vi "LED Controller.vi"(8 "error in":errorcluster) -> ()   [LabVIEW 2023]
doc: "This VI executes continuously carrying out the current operation and responding to updates or new operations. It will often contain the timing or control code that is difficult to place directly in TeleOp. This VI generally opens all sensors and motors and isolates the rest of the robot code from knowing how the operations are carried out."
uses:
  <vilib>/Rock Robotics/WPI/Framework/Completion Status.ctl
  LED Setpoints.ctl
  LED Operations.ctl
  source files/Amp-Speaker.ctl
  source files/Lights Setpoints.ctl
  <vilib>/Rock Robotics/SystemInterfaces/DIO/FPGA_DIOPWMChannel.ctl
  source files/ArduinoSerialBling.lvlib
  <vilib>/Rock Robotics/Network Tables/NT Write Boolean.vi
panel:
  in  "Blending LEDs":u8=21
  in  "String Length":u16=21
  in  "Interactive Values":T1
  out "Current\nCmd":string
  in  "Buttons":cluster{"Execute Cmd":bool, "Abort Cmd":bool}
  out "Command Timing":cluster{"Start Time (ms)":u32, "Iterations":i32}
  out "Status":T5
  # "Tip: It may be helpful to observe inputs and sensor values.\nYou may also want to display tuning or debugging controls."
  # "Interactive Command: You may fill in the settings for a command\nand schedule it with the Execute button. You can observe and abort\nany command while fine tuning the code for the controller."
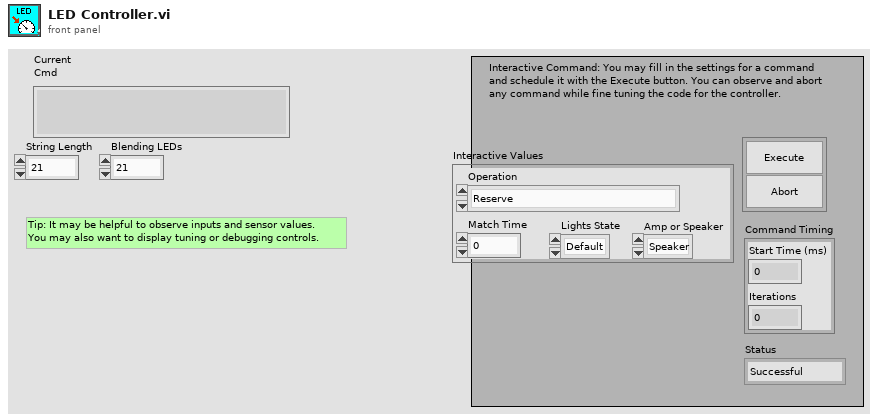
[diagram p1: front panel]
types:
  T1 = typedef "LED Setpoints.ctl" = cluster{"Operation":T2, "Match Time":dbl, "Lights State":T3, "Amp or Speaker":T4}
  T2 = typedef "LED Operations.ctl" = enum16{"Reserve", "Read Current", "Immediate"}
  T3 = typedef "Amp-Speaker.ctl" = enum16{"Default", "Flywheel State", "Endgame", "Note Detection"}
  T4 = typedef "Lights Setpoints.ctl" = enum16{"Speaker", "Amp"}
  T5 = typedef "Completion Status.ctl" = enum16{"Successful", "Aborted", "Incomplete"}
  T6 = typedef "FPGA_DIOPWMChannel.ctl" = enum8{"PWM 0", "PWM 1", "PWM 2", "PWM 3", "PWM 4", "PWM 5", "PWM 6", "PWM 7", "PWM 8", "PWM 9", "PWM MXP 0", "PWM MXP 1", "PWM MXP 2", "PWM MXP 3", "PWM MXP 4", "PWM MXP 5", "PWM MXP 6", "PWM MXP 7", "PWM MXP 8", "PWM MXP 9", "Invalid"}
  T7 = typedef "WPI_PWMDeviceRef.ctl" = cluster{"DeviceStatus":errorcluster, "PWM Channel":T6}
  T8 = typedef "Command Status Info.ctl" = cluster{"Name":string, "Status":T5, "notifier out":T9}
  T9 = typedef "Completion Notifier.ctl" = refnum<notifier>
  T10 = cluster{"Current Command":T1, "Command Timing":cluster{"Start Time (ms)":u32, "Iterations":i32}, "Command Arguments":cluster{"Command Info":T8, "Description":string, "Default Command":T1, "queue out":refnum<queue>, "Subsystem Name":string}}
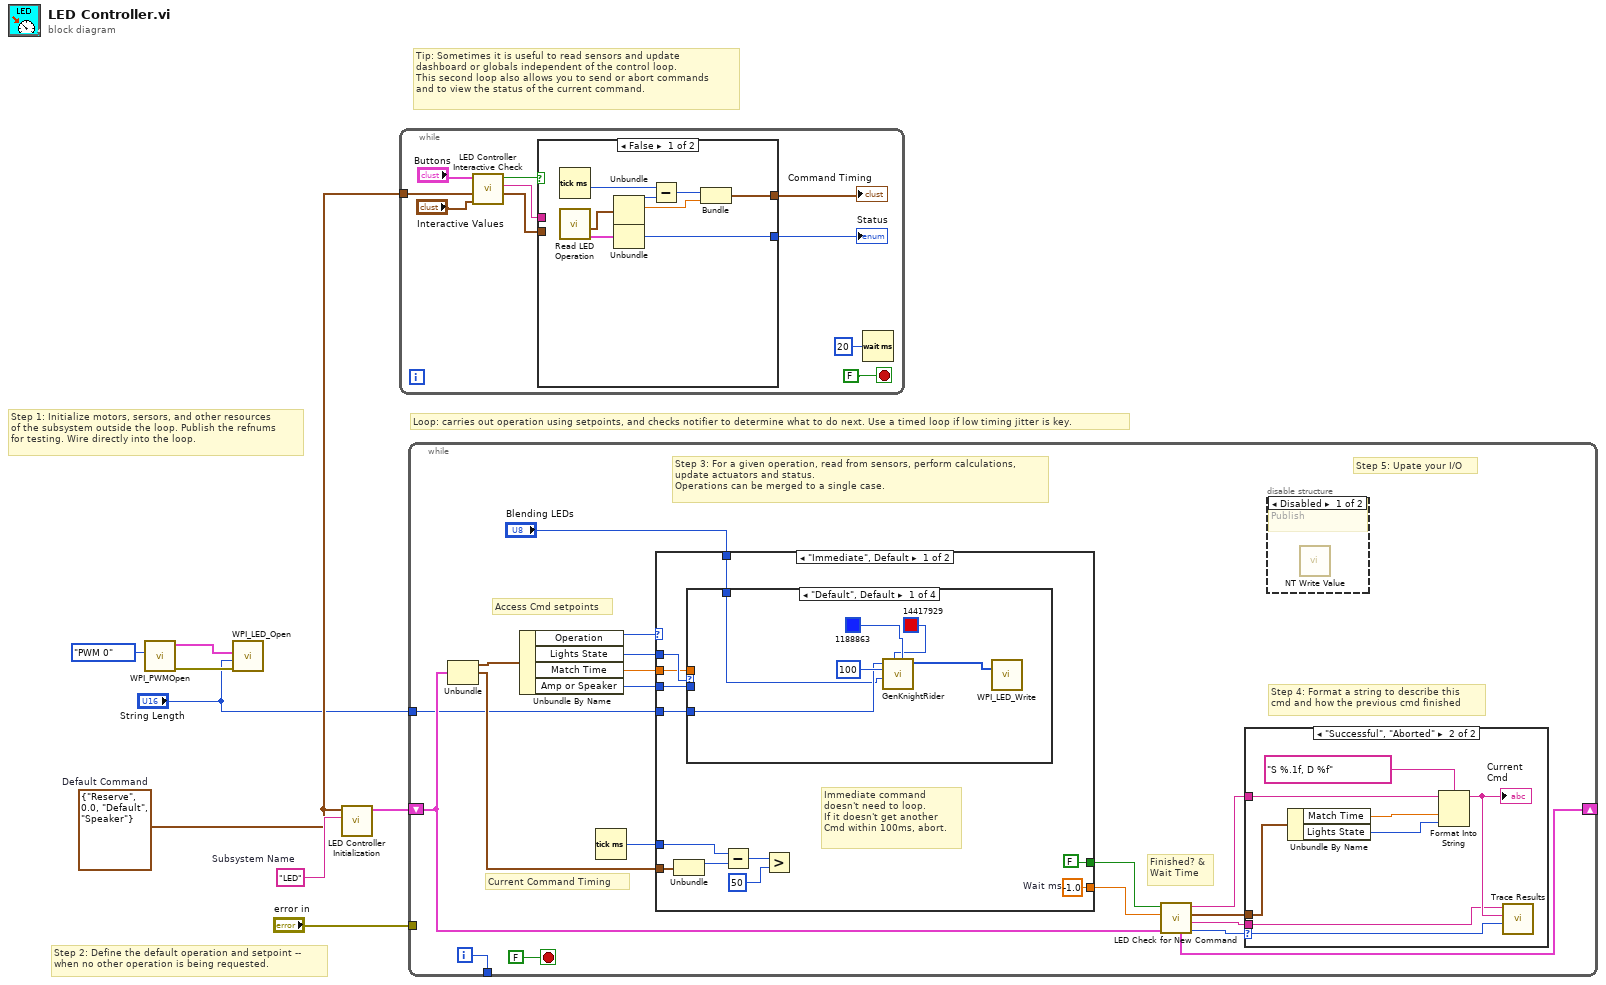
[diagram p0: block diagram]
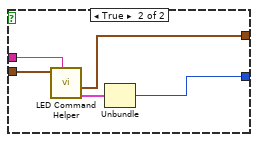
[diagram p2: hidden frame]
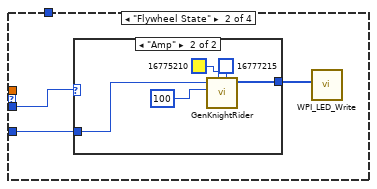
[diagram p5: hidden frame]
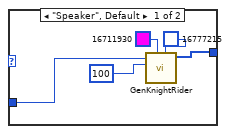
[diagram p6: hidden frame]
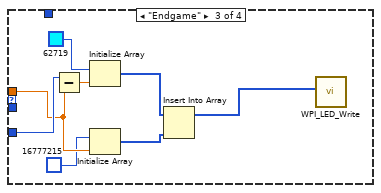
[diagram p7: hidden frame]
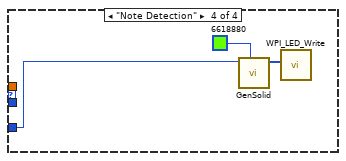
[diagram p8: hidden frame]
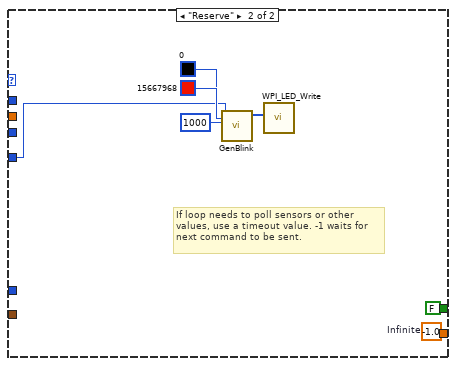
[diagram p9: hidden frame]
diagram:
  w5 = T1 {"Operation"=enum."Reserve", "Match Time"=0.0, "Lights State"=enum."Default", "Amp or Speaker"=enum."Speaker"}  # Default Command
  w6 = "LED"  # Subsystem Name
  # "Tip: Sometimes it is useful to read sensors and update\ndashboard or globals independent of the control loop.\nThis second loop also allows you to send or abort commands\nand to view the status of the current command."
  # "Step 2: Define the default operation and setpoint --\nwhen no other operation is being requested."
  # "Step 1: Initialize motors, sersors, and other resources\nof the subsystem outside the loop. Publish the refnums\nfor testing. Wire directly into the loop."
  # "Loop: carries out operation using setpoints, and checks notifier to determine what to do next. Use a timed loop if low timing jitter is key."
  n1 = call <vilib>:"WPI_PWMOpen.vi"("PWM Channel"=FPGA_DIOPWMChannel."PWM 0") -> ("error out"=w2:errorcluster, "PWMDeviceRef"=w3:T7)  [unwired: 9 in]
  n2 = call <vilib>:"WPI_LED_Open.vi"("error in"=w2, "String Length"="String Length", "PWMDeviceRef"=w3) -> ()  [unwired: 8 in, 1 out]
  n3 = call "LED Controller Initialization.vi"("Subsystem Name"=w6, "Default Command"=w5) -> ("Current Command"=w7:T10)  [unwired: 9 in]
  n4 = while {
    tunnel: w5 -> [w15]
    stop <- FALSE stop-if-true
    n5 = call "LED Controller Interactive Check.vi"("Interactive Command in"="Interactive Values", "Default Command"=w15, "Buttons"="Buttons") -> ("Interactive Command out"=w12:T1, "Trace String"=w13:string, "Schedule"=w14:bool)  [unwired: 6 in]
    n6 = case shown="False" w14 {
      tunnel: [w26 w31] -> w11
      tunnel: w12 -> [_ w29]
      tunnel: [w22 w27] -> w10
      tunnel: w13 -> [_ w30]
      frame False {
        n7 = Tick Count (ms)() -> (millisecond timer value=w21:u32)
        n8 = call "Read LED Operation.vi"() -> ("Command Info"=w19:T8, "SubSystem Data"=w20:T1)  [unwired: 9 in, 1 out]
        n9 = Unbundle(w20) -> ("Operation"=w25:T2, "Match Time"=w23:dbl)  [unwired: 2 out]
        n10 = Unbundle(w19) -> ("Status"=w26:T5)  [unwired: 2 out]
        n11 = Subtract(x=w21, y=w25) -> (x-y=w24:u32)
        n12 = Bundle(w24, "Match Time"=w23) -> (w22:cluster{u32, "Match Time":dbl})  [unwired: 1 in]
      }
      frame True {
        n13 = call "LED Command Helper.vi"("Description"=w30, "SubSystem Data"=w29) -> ("Command Info Out"=w28:T8, "Command Timing"=w27:cluster{"Start Time (ms)":u32, "Iterations":i32})  [unwired: 7 in, 1 out]
        n14 = Unbundle(w28) -> ("Status"=w31:T5)  [unwired: 2 out]
      }
    }
    "Status" <- w11
    "Command Timing" <- w10
    n15 = Wait (ms)(milliseconds to wait=u32 20) -> ()  [unwired: 1 out]
  }
  n16 = while {
    shift-right: [w42] -> _
    shift-left: w7 -> [w35]
    tunnel: [w49] -> _
    tunnel: "error in" -> [_]
    tunnel: "String Length" -> [w34]
    i -> [w49]
    stop <- FALSE stop-if-true
    # "Step 5: Upate your I/O"
    # "Step 4: Format a string to describe this\ncmd and how the previous cmd finished"
    # "Current Command Timing"
    # "Access Cmd setpoints"
    # "Finished? &\nWait Time"
    # "Step 3: For a given operation, read from sensors, perform calculations,\nupdate actuators and status.\nOperations can be merged to a single case."
    n17 = Unbundle(w35) -> ("Current Command"=w48:T1, "Command Timing"=w44:cluster{"Start Time (ms)":u32, "Iterations":i32})  [unwired: 1 out]
    n18 = Unbundle By Name(w48) -> ("Operation"=w47:T2, "Lights State"=w46:T3, "Match Time"=w43:dbl, "Amp or Speaker"=w33:T4)
    n19 = Tick Count (ms)() -> (millisecond timer value=w45:u32)
    n20 = case shown="\"Immediate\", Default" w47 {
      tunnel: [w70 w107] -> w40
      tunnel: [FALSE ("ignore previous (F)") FALSE ("ignore previous (F)")] -> w41
      tunnel: w44 -> [w66 _]
      tunnel: w46 -> [w64 _]
      tunnel: w45 -> [w65 _]
      tunnel: w43 -> [w62 _]
      tunnel: w34 -> [w63 w102]
      tunnel: w33 -> [w60 _]
      tunnel: "Blending LEDs" -> [w59 _]
      frame "Immediate", Default {
        w70 = -1.0  # Wait ms
        # "Immediate command\ndoesn't need to loop.\nIf it doesn't get another\nCmd within 100ms, abort."
        n21 = Unbundle(w66) -> ("Start Time (ms)"=w69:u32)  [unwired: 1 out]
        n22 = case shown="\"Default\", Default" w64 {
          tunnel: w63 -> [w72 w79 w97 w100]
          tunnel: w62 -> [_ _ w95 _]
          tunnel: w60 -> [_ w78 _ _]
          tunnel: w59 -> [w71 _ _ _]
          frame "Default", Default {
            n23 = call "GenKnightRider.vi"("Background Color"=u32 1188863, "Foreground Color"=u32 14417929, "Blending LEDs"=w71, "Sine Rate"=100, "NumLeds"=w72) -> ("Array"=w76:u32[])  [unwired: 5 in, 1 out]
            n24 = call <vilib>:"WPI_LED_Write.vi"("Color Array"=w76) -> ()  [unwired: 10 in, 1 out]
          }
          frame "Flywheel State" {
            n25 = case shown="\"Amp\"" w78 {
              tunnel: w79 -> [w80 w88]
              tunnel: [w81 w85] -> w77
              frame "Speaker", Default {
                n26 = call "GenKnightRider.vi"("Background Color"=u32 16777215, "Foreground Color"=u32 16711930, "Sine Rate"=100, "NumLeds"=w80) -> ("Array"=w81:u32[])  [unwired: 6 in, 1 out]
              }
              frame "Amp" {
                n27 = call "GenKnightRider.vi"("Background Color"=u32 16777215, "Foreground Color"=u32 16775210, "Sine Rate"=100, "NumLeds"=w88) -> ("Array"=w85:u32[])  [unwired: 6 in, 1 out]
              }
            }
            n28 = call <vilib>:"WPI_LED_Write.vi"("Color Array"=w77) -> ()  [unwired: 10 in, 1 out]
          }
          frame "Endgame" {
            n29 = Subtract(x=w97, y=w95) -> (x-y=w96:dbl)
            n30 = Initialize Array(u32 62719, w96) -> (w91:u32[])
            n31 = Initialize Array(u32 16777215, w95) -> (w92:u32[])
            n32 = Insert Into Array(array=w91, new element=w92) -> (w90:u32[])  [unwired: 1 in]
            n33 = call <vilib>:"WPI_LED_Write.vi"("Color Array"=w90) -> ()  [unwired: 10 in, 1 out]
          }
          frame "Note Detection" {
            n34 = call "GenSolid.vi"("Color"=u32 6618880, "NumLeds"=w100) -> ("Array"=w98:u32[])  [unwired: 9 in]
            n35 = call <vilib>:"WPI_LED_Write.vi"("Color Array"=w98) -> ()  [unwired: 10 in, 1 out]
          }
        }
        n36 = Subtract(x=w65, y=w69) -> (x-y=w68:u32)
        n37 = Greater?(x=w68, y=u8 50 ("Left Motor")) -> ()  [unwired: 1 out]
      }
      frame "Reserve" {
        w107 = -1.0  # Infinite
        # "If loop needs to poll sensors or other\nvalues, use a timeout value. -1 waits for\nnext command to be sent."
        n38 = call "GenBlink.vi"("Color 2"=u32 0, "Color 1"=u32 15667968, "Period (ms)"=1000 ("Sine Rate"), "NumLeds"=w102) -> ("Array"=w101:u32[])  [unwired: 6 in, 1 out]
        n39 = call <vilib>:"WPI_LED_Write.vi"("Color Array"=w101) -> ()  [unwired: 10 in, 1 out]
      }
    }
    n40 = call "LED Check for New Command.vi"("Current Command"=w35, "Wait time (ms)"=w40, "Finished?"=w41) -> ("Completion"=w36:T5, "Subsystem Name"=w37:string, "Current Command"=w38:T1, "Initial Trace String"=w39:string, "NextCommand"=w42:T10)  [unwired: 4 in]
    n41 = case shown="\"Successful\", \"Aborted\"" w36 {
      selector: w36 -> [_ w58]
      tunnel: w39 -> [_ w54]
      tunnel: w38 -> [_ w55]
      tunnel: w37 -> [_ w51]
      frame "Incomplete", Default {
        # "Continuing current command"
      }
      frame "Successful", "Aborted" {
        # "Report and setup for next command"
        n42 = Unbundle By Name(w55) -> ("Match Time"=w57:dbl, "Lights State"=w52:T3)
        n43 = Format Into String(format string="S %.1f, D %f", initial string=w54, w57, w52) -> (resulting string=w53:string)  [unwired: 1 in, 1 out]
        "Current\nCmd" <- w53
        n44 = call <vilib>:"Trace Results.vi"("Status of previous command"=w58, "Description"=w53, "Subsystem"=w51) -> ()  [unwired: 9 in]
      }
    }
    n45 = disable-structure shown="Disabled" {
      frame Disabled {
        # "Publish"
        n46 = call-poly <vilib>:"NT Write Value.vi"() -> ()  [unwired: 11 in, 1 out]
      }
      frame Enabled {
      }
    }
  }
